vi "VoltageDebug.vi"(8 "delay (ms)":u32=500) -> ()   [LabVIEW 2013]
panel:
  out "Array of Voltages":string[](array[string])
  in  "VISA PS":refnum<visa-resource-name>="COM1"
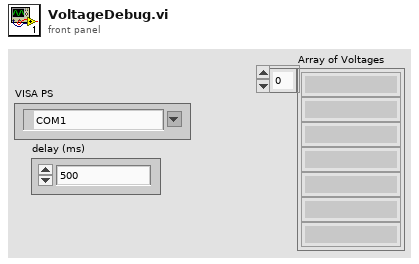
[diagram p1: front panel]
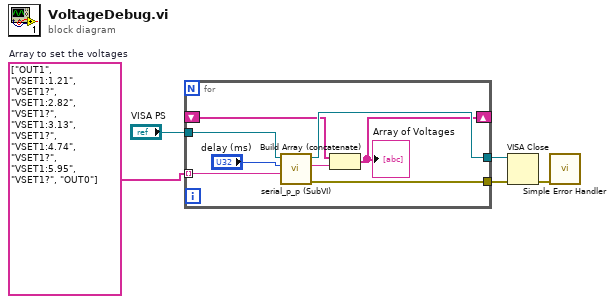
[diagram p0: block diagram]
diagram:
  w3 = string[] ["OUT1", "VSET1:1.21", "VSET1?", "VSET1:2.82", "VSET1?", "VSET1:3.13", "VSET1?", "VSET1:4.74", "VSET1?", "VSET1:5.95", "VSET1?", "OUT0"]  # Array to set the voltages
  n1 = for {
    tunnel: "VISA PS" -> [w12]
    tunnel: w3 -> [w11] mode=indexing
    tunnel: [w8] -> w4
    tunnel: [w9] -> w2
    shift-right: [w6] -> _
    shift-left: _ -> [w7]
    n2 = call "serial_p_p (SubVI).vi"("Command"=w11, "delay before read (ms)"="delay (ms)", "VISA Refnum in"=w12) -> ("error out"=w9:errorcluster, "read buffer"=w10:string, "VISA Refnum out"=w8:refnum<visa-resource-name>)  [unwired: 6 in]
    n3 = Build Array (concatenate)(w7, w10) -> (w6:string[])
    "Array of Voltages" <- w6
  }
  n4 = VISA Close(VISA resource name=w4, error in (no error)=w2) -> (error out=w1:errorcluster)
  n5 = call <vilib>:"Simple Error Handler.vi"("error in (no error)"=w1) -> ()  [unwired: 4 in, 5 out]
